vi "EngTeacher_Main.vi"() -> ()   [LabVIEW 2020]
uses:
  #typedef_TeacherDataBase.ctl
  #typedef_LearnigAction.ctl
panel:
  out "English":string
  out "Polish":string
  in  "Exit":bool
  in  "Stop":bool
  in  "Start Test":bool
  in  "Start Learning":bool
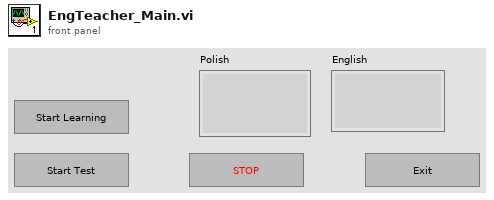
[diagram p1: front panel]
types:
  T1 = typedef "#typedef_LearnigAction.ctl" = enum16{"Empty", "English Word", "Polish Word"}
  T2 = typedef "#typedef_TeacherDataBase.ctl" = cluster{"English":path, "Polish":path}
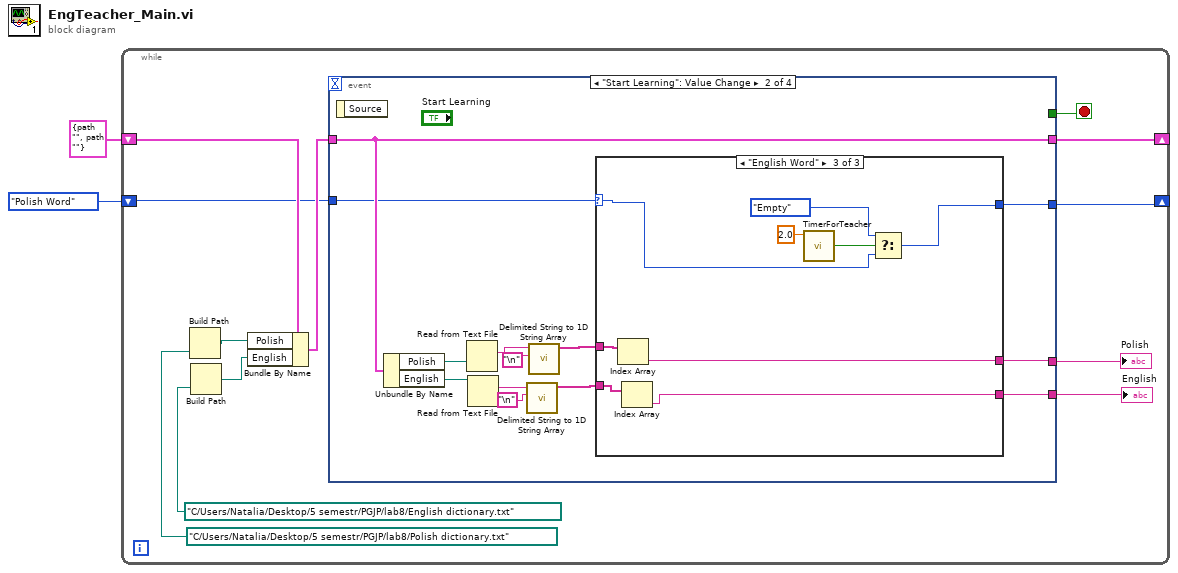
[diagram p0: block diagram]
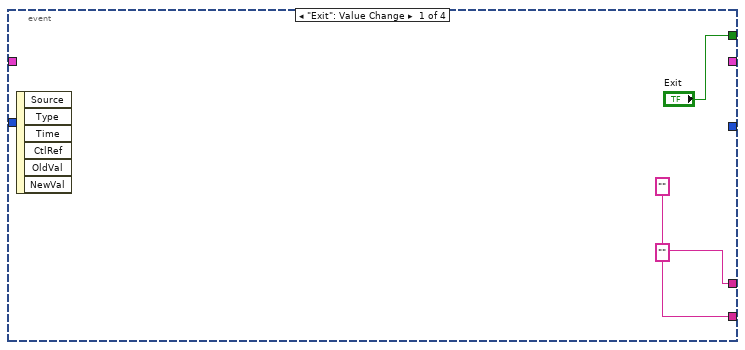
[diagram p2: hidden frame]
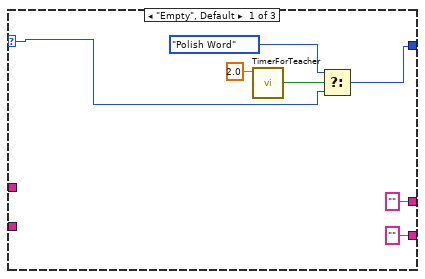
[diagram p3: hidden frame]
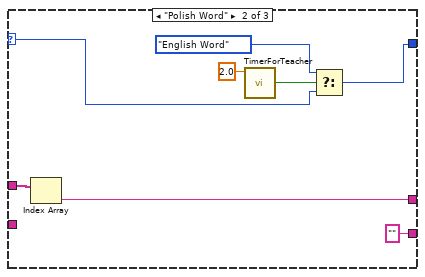
[diagram p4: hidden frame]
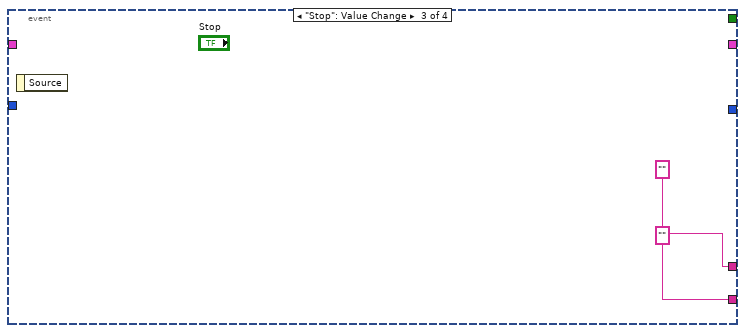
[diagram p5: hidden frame]
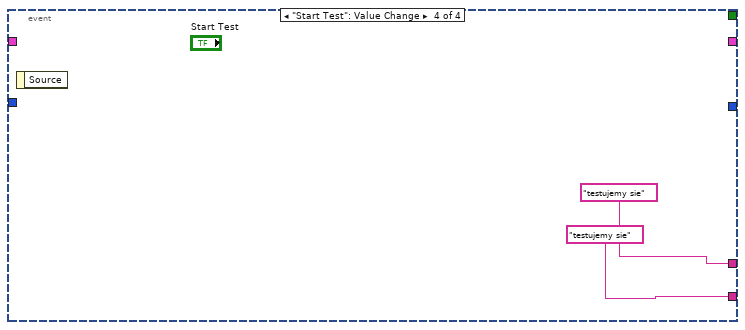
[diagram p6: hidden frame]
diagram:
  n1 = while {
    shift-right: [w11] -> _
    shift-left: T2 {"English"=path "", "Polish"=path ""} ("Data Base") -> [w10]
    shift-right: [w3] -> _
    shift-left: #typedef_LearnigAction."Polish Word" ("Learning Action") -> [w4]
    stop <- w14 stop-if-true
    n2 = Build Path(name or relative path=path "C:/Users/Natalia/Desktop/5 semestr/PGJP/lab8/Polish dictionary.txt") -> (appended path=w8:path)  [unwired: 1 in]
    n3 = Build Path(name or relative path=path "C:/Users/Natalia/Desktop/5 semestr/PGJP/lab8/English dictionary.txt") -> (appended path=w7:path)  [unwired: 1 in]
    n4 = Bundle By Name(cluster=w10, "Polish"=w8, "English"=w7) -> (w9:T2)
    n5 = event shown="[1] \"Start Learning\": Value Change" {
      selector: _ -> [_ _ _ _]
      dyn-events: _ -> [_ _ _ _]
      timeout: _ -> [_ _ _ _]
      tunnel: ["Exit" _ _ _] -> w14
      tunnel: ["" ("English") w22 "" ("English") "testujemy sie" ("English")] -> w13
      tunnel: ["" ("Polish") w24 "" ("Polish") "testujemy sie" ("Polish")] -> w12
      tunnel: w9 -> [_ w25 _ _]
      tunnel: [_ w25 _ _] -> w11
      tunnel: w4 -> [_ w19 _ _]
      tunnel: [_ w18 _ _] -> w3
      event "Exit": Value Change {
        n6 = event-data() -> ()  [unwired: 1 in, 6 out]
      }
      event "Start Learning": Value Change {
        n7 = event-data() -> ()  [unwired: 1 in, 1 out]
        n8 = Unbundle By Name(w25) -> ("Polish"=w30:path, "English"=w29:path)
        n9 = Read from Text File(file (use dialog)=w30) -> (text=w27:string)  [unwired: 3 in, 3 out]
        n10 = Read from Text File(file (use dialog)=w29) -> (text=w28:string)  [unwired: 3 in, 3 out]
        n11 = call <vilib>:"Delimited String to 1D String Array.vi"("delimiter"="\n", "delimited string"=w28) -> ("string array"=w23:string[])  [unwired: 9 in]
        n12 = call <vilib>:"Delimited String to 1D String Array.vi"("delimiter"="\n", "delimited string"=w27) -> ("string array"=w26:string[])  [unwired: 9 in]
        n13 = case shown="\"English Word\"" w19 {
          selector: w19 -> [w32 w38 w47]
          tunnel: w26 -> [_ w45 w54]
          tunnel: ["" ("String") w44 w53] -> w24
          tunnel: w23 -> [_ _ w52]
          tunnel: ["" ("String") "" ("String") w51] -> w22
          tunnel: [w31 w39 w46] -> w18
          frame "Empty", Default {
            n14 = call "TimerForTeacher.vi"("Time to Elapse (2s)"=2.0) -> ("Time Elapsed?"=w35:bool)  [unwired: 8 in, 2 out]
            n15 = Select(t=#typedef_LearnigAction."Polish Word" ("Learning Action"), s=w35, f=w32) -> (s? t:f=w31:T1)
          }
          frame "Polish Word" {
            n16 = Index Array(array=w45) -> (element=w44:string)  [unwired: 1 in]
            n17 = call "TimerForTeacher.vi"("Time to Elapse (2s)"=2.0) -> ("Time Elapsed?"=w42:bool)  [unwired: 8 in, 2 out]
            n18 = Select(t=#typedef_LearnigAction."English Word" ("Learning Action"), s=w42, f=w38) -> (s? t:f=w39:T1)
          }
          frame "English Word" {
            n19 = Index Array(array=w54) -> (element=w53:string)  [unwired: 1 in]
            n20 = Index Array(array=w52) -> (element=w51:string)  [unwired: 1 in]
            n21 = call "TimerForTeacher.vi"("Time to Elapse (2s)"=2.0) -> ("Time Elapsed?"=w50:bool)  [unwired: 8 in, 2 out]
            n22 = Select(t=#typedef_LearnigAction."Empty" ("Learning Action"), s=w50, f=w47) -> (s? t:f=w46:T1)
          }
        }
      }
      event "Stop": Value Change {
        n23 = event-data() -> ()  [unwired: 1 in, 1 out]
      }
      event "Start Test": Value Change {
        n24 = event-data() -> ()  [unwired: 1 in, 1 out]
      }
    }
    "English" <- w13
    "Polish" <- w12
  }
